vi "PicoLog1000ExampleStreaming.vi"(1 "stop":bool) -> ()   [LabVIEW 2010]
panel:
  out "UnitInfo":T1
  out "maxValue":u16
  in  "Apply":bool
  in  "Duty Cycle (%)":u8 max=100
  in  "Period (microseconds)":u16=100 min=100 max=1800
  in  "D3":bool=TRUE
  in  "D2":bool=TRUE
  in  "D1":bool=TRUE
  in  "D0":bool=TRUE
  in  "Trigger":T2={"Enabled"=FALSE, "AutoTrigger"=FALSE, "delay (%)"=-50.0, "Auto Trigger\nTiime (ms)"=1000, "Channel"=1, "Trigger Direction"=0, "threshold (mV)"=500, "hysteresis (mV)"=5} {"Trigger Direction" items=["rising edge", "falling edge"]; "Channel" items=["Ch1"=1, "Ch2"=2, "Ch3"=3, "Ch4"=4, "Ch5"=5, "Ch6"=6, "Ch7"=7, "Ch8"=8, "Ch9"=9, "Ch10"=10, "Ch11"=11, "Ch12"=12, "Ch13"=13, "Ch14"=14, "Ch15"=15, "Ch16"=16]}
  out "Ch Over Range":bool[](array[boolean])
  out "Ready":bool
  out "pl1000 handle out":i16
  out "error out":errorcluster
  in  "error in (no error)":errorcluster
  out "noOfValues":u32
  out "Triggered":bool
  out "Sampling rate (S/s)":dbl
  out "No. of channels":i16=12
  in  "Channels Enabled":string="1,2,3,4,5,6,7,8,9,10,11,12"
  out "Waveform Chart":dbl[][](graph)
  in  "Desired sample rate (S/s)":u32=2000 max=100000
  # "Streaming Mode Example"
  # "(e.g. 1,2,3)"
  # "Digital Outputs"
  # "Pulse-Width Modulation"
  # "OFF"
  # "ON"
  # "Trigger delay of \n-50% means the\ntrigger event is\nin the middle of \nthe block"
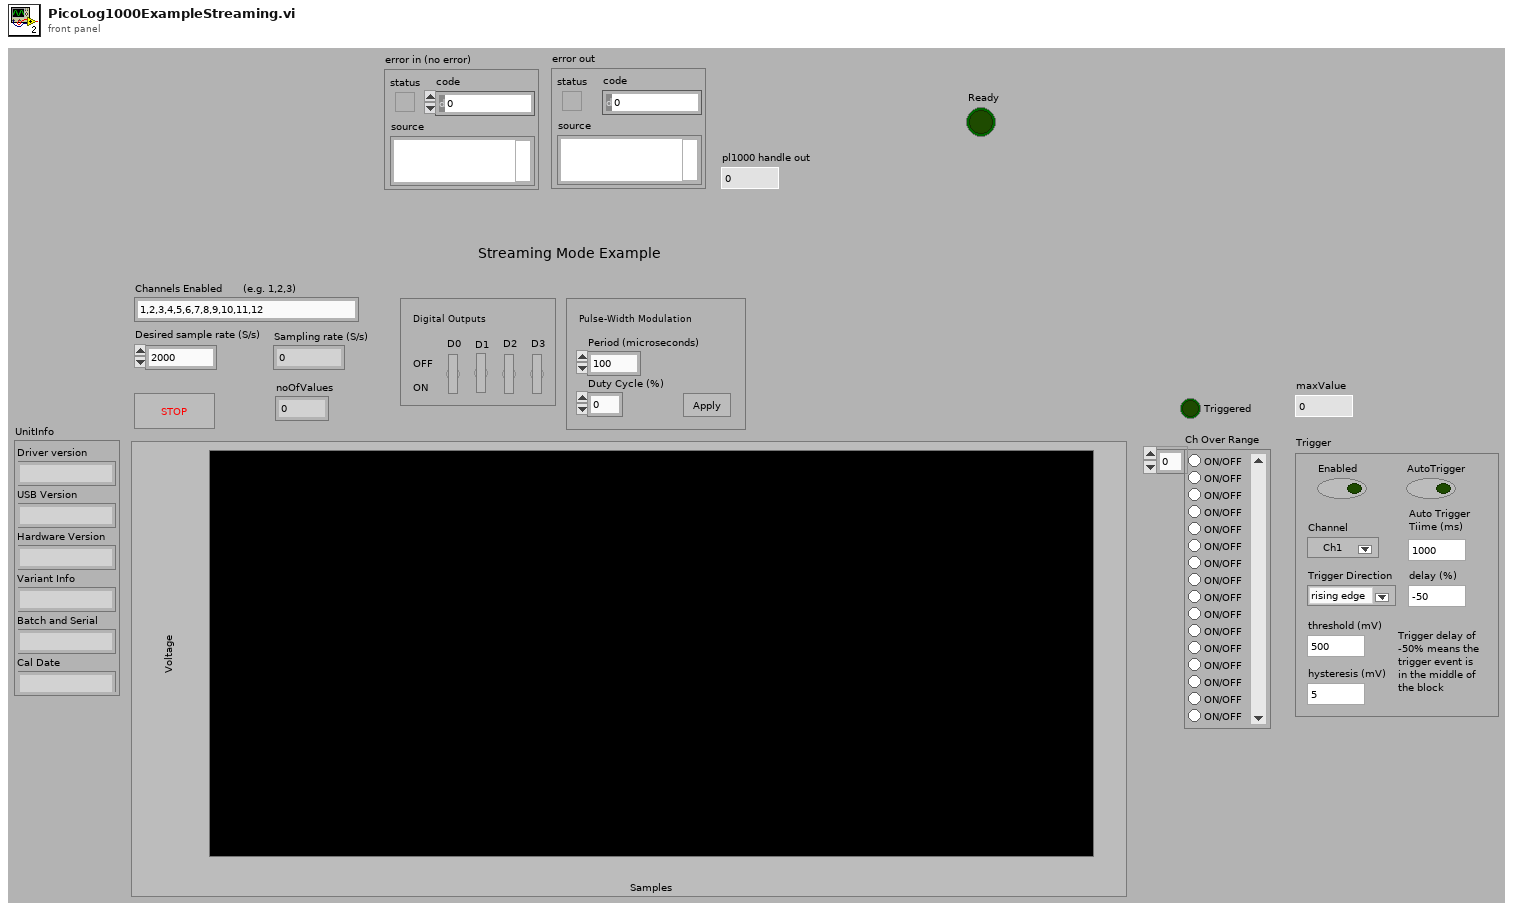
[diagram p1: front panel]
types:
  T1 = cluster{"Driver version":string, "USB Version":string, "Hardware Version":string, "Variant Info":string, "Batch and Serial":string, "Cal Date":string, "[6]":string, "[7]":string, "[8]":string}
  T2 = cluster{"Enabled":bool, "AutoTrigger":bool, "delay (%)":sgl, "Auto Trigger\nTiime (ms)":u16, "Channel":u16, "Trigger Direction":u16, "threshold (mV)":u16, "hysteresis (mV)":u16}
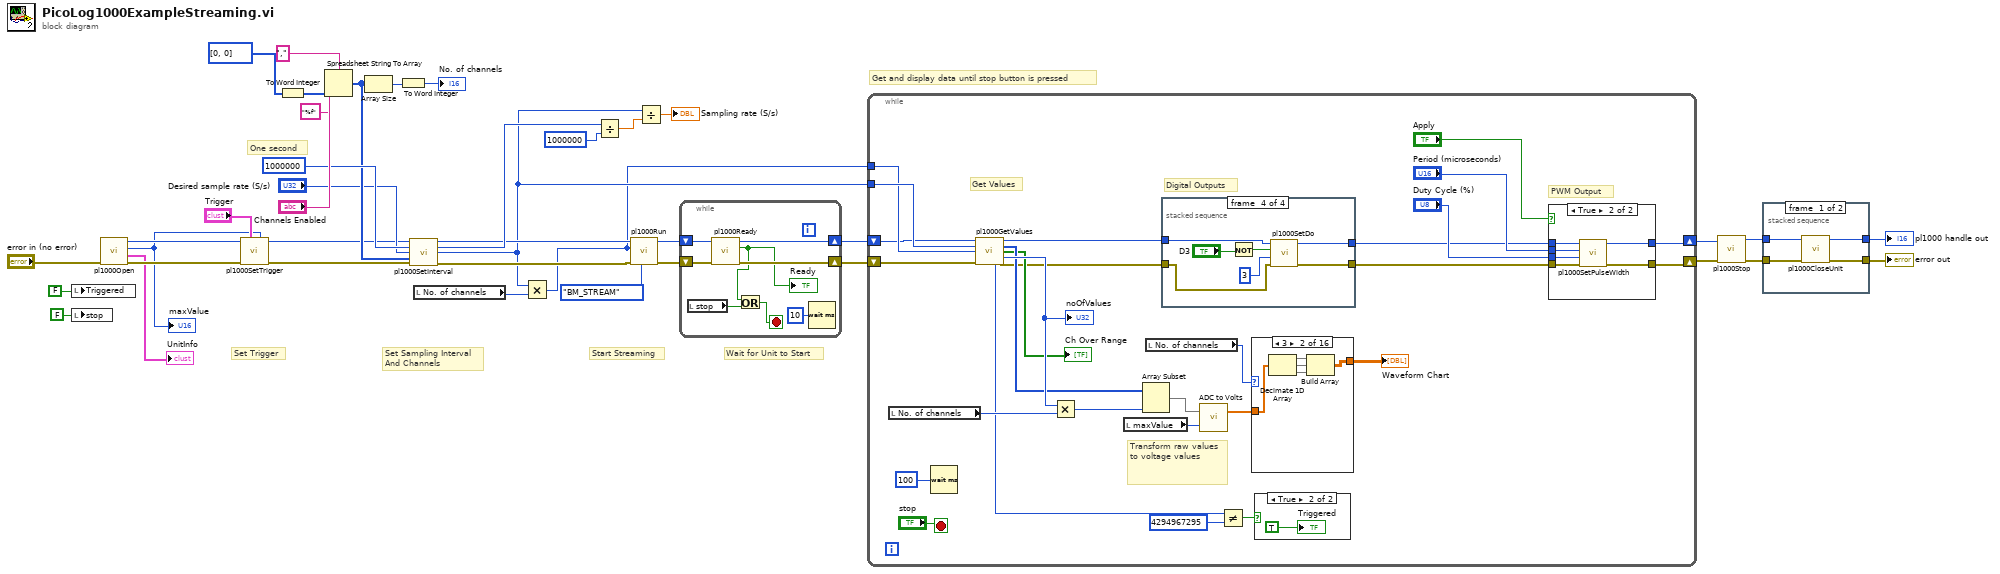
[diagram p0: block diagram]
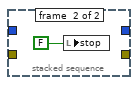
[diagram p2: hidden frame]
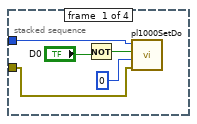
[diagram p4: hidden frame]
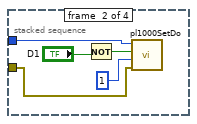
[diagram p5: hidden frame]
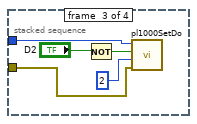
[diagram p6: hidden frame]
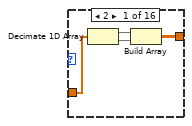
[diagram p8: hidden frame]
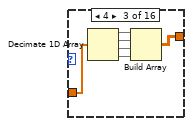
[diagram p9: hidden frame]
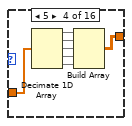
[diagram p10: hidden frame]
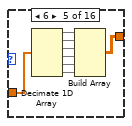
[diagram p11: hidden frame]
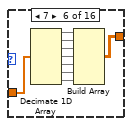
[diagram p12: hidden frame]
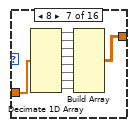
[diagram p13: hidden frame]
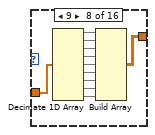
[diagram p14: hidden frame]
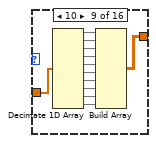
[diagram p15: hidden frame]
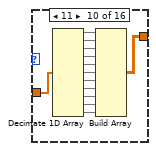
[diagram p16: hidden frame]
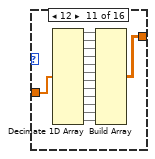
[diagram p17: hidden frame]
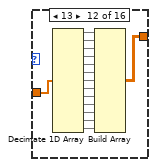
[diagram p18: hidden frame]
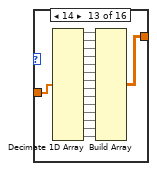
[diagram p19: hidden frame]
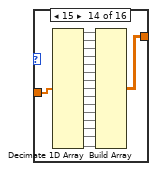
[diagram p20: hidden frame]
diagram:
  # "Wait for Unit to Start"
  # "Start Streaming"
  # "Set Sampling Interval\nAnd Channels"
  # "Set Trigger"
  # "Get and display data until stop button is pressed"
  # "One second"
  n1 = local write "Triggered"(FALSE ("Boolean")) -> ()
  n2 = local write "stop"(FALSE ("stop")) -> ()
  n3 = call "pl1000Open.vi"("error in (no error)"="error in (no error)") -> ("error out"=w11:errorcluster, "UnitInfo"=→"UnitInfo":T1, "maxValue"=w2:u16, "pl1000 handle out"=w7:i16)  [unwired: 7 in]
  "maxValue" <- w2
  n4 = call "pl1000SetTrigger.vi"("pl1000 handle"=w7, "Trigger"="Trigger", "maxValue"=w2, "error in (no error)"=w11) -> ("pl1000 handle out"=w9:i16, "error out"=w10:errorcluster)  [unwired: 10 in]
  n5 = To Word Integer(number=u32[] [0, 0] ("array type (2D Dbl)")) -> (16bit integer=w30:i16[])
  n6 = Spreadsheet String To Array(delimiter (Tab)=",", format string="%f", spreadsheet string="Channels Enabled", array type (2D Dbl)=w30) -> (array=w26:i16[])
  n7 = Array Size(array=w26) -> (size(s)=w32:i32)
  n8 = To Word Integer(number=w32) -> (16bit integer=→"No. of channels":i16)
  n9 = call "pl1000SetInterval.vi"("pl1000 handle"=w9, "usForBlock"=u32 1000000 ("us_for_block"), "idealNoOfSamples"="Desired sample rate (S/s)", "channels"=w26, "error in (no error)"=w10) -> ("pl1000 handle out"=w22:i16, "usForBlock OP"=w25:u32, "idealNoOfSamples OP"=w17:u32, "error out"=w23:errorcluster)  [unwired: 7 in]
  n10 = local read "No. of channels"() -> (w35:i16)
  n11 = Multiply(x=w17, y=w35) -> (x*y=w16:u32)
  n12 = Divide(x=w25, y=u32 1000000) -> (x/y=w36:dbl)
  n13 = call "pl1000Run.vi"("method"=enum16{"BM_SINGLE", "BM_WINDOW", "BM_STREAM"}."BM_STREAM", "error in (no error)"=w23, "noOfValues"=w16, "pl1000 handle"=w22) -> ("error out"=w20:errorcluster, "pl1000 handle out"=w19:i16)  [unwired: 6 in]
  n14 = Divide(x=w17, y=w36) -> (x/y=→"Sampling rate (S/s)":dbl)
  n15 = while {
    shift-right: [w46] -> w18
    shift-left: w19 -> [w48]
    shift-right: [w45] -> w15
    shift-left: w20 -> [w47]
    stop <- w43 stop-if-true
    n16 = local read "stop"() -> (w41:bool)
    n17 = call "pl1000Ready.vi"("error in (no error)"=w47, "pl1000 handle"=w48) -> ("error out"=w45:errorcluster, "ready"=w42:bool, "pl1000 handle out"=w46:i16)  [unwired: 7 in]
    "Ready" <- w42
    n18 = Or(x=w42, y=w41) -> (x .or. y?=w43:bool)
    n19 = Wait (ms)(milliseconds to wait=u32 10) -> ()  [unwired: 1 out]
  }
  n20 = while {
    tunnel: w17 -> [w66]
    tunnel: w16 -> [w65]
    shift-right: [w51] -> w13
    shift-left: w15 -> [w61]
    shift-right: [w50] -> w12
    shift-left: w18 -> [w59]
    stop <- "stop" stop-if-true
    # "Transform raw values to voltage values"
    # "Get Values"
    # "PWM Output"
    # "Digital Outputs"
    n21 = local read "No. of channels"() -> (w73:i16)
    n22 = Wait (ms)(milliseconds to wait=u32 100) -> ()  [unwired: 1 out]
    n23 = call "pl1000GetValues.vi"("pl1000 handle"=w59, "noOfValues"=w66, "SizeOfArray"=w65, "error in (no error)"=w61) -> ("pl1000 handle out"=w58:i16, "values"=w67:u16[], "Ch Over Range"=→"Ch Over Range":bool[], "noOfValues collected per ch"=w68:u32, "triggerIndex"=w64:u32, "error out"=w57:errorcluster)  [unwired: 6 in]
    "noOfValues" <- w68
    n24 = Multiply(x=w68, y=w73) -> (x*y=w72:u32)
    n25 = local read "maxValue"() -> (w49:u16)
    n26 = Array Subset(array=w67, length=w72) -> (w63:u16[])  [unwired: 1 in]
    n27 = local read "No. of channels"() -> (w75:i16)
    n28 = stacked-sequence {
      tunnel: w58 -> [w86 w91 w96 w103]
      tunnel: w57 -> [w85 w90 w95 w100]
      tunnel: [_ _ _ w101] -> w52
      tunnel: [_ _ _ w102] -> w53
      frame #0 {
        n29 = Not(x="D0") -> (.not. x?=w89:bool)
        n30 = call "pl1000SetDo.vi"("error in (no error)"=w85, "DO Channel"=0, "DO State"=w89, "pl1000 handle"=w86) -> ()  [unwired: 6 in, 2 out]
      }
      frame #1 {
        n31 = Not(x="D1") -> (.not. x?=w94:bool)
        n32 = call "pl1000SetDo.vi"("error in (no error)"=w90, "DO Channel"=1, "DO State"=w94, "pl1000 handle"=w91) -> ()  [unwired: 6 in, 2 out]
      }
      frame #2 {
        n33 = Not(x="D2") -> (.not. x?=w99:bool)
        n34 = call "pl1000SetDo.vi"("error in (no error)"=w95, "DO Channel"=2, "DO State"=w99, "pl1000 handle"=w96) -> ()  [unwired: 6 in, 2 out]
      }
      frame #3 {
        n35 = Not(x="D3") -> (.not. x?=w106:bool)
        n36 = call "pl1000SetDo.vi"("error in (no error)"=w100, "DO Channel"=3, "DO State"=w106, "pl1000 handle"=w103) -> ("error out"=w101:errorcluster, "pl1000 handle out"=w102:i16)  [unwired: 6 in]
      }
    }
    n37 = call "ADC to Volts.vi"("maxValue"=w49, "ADC values"=w63) -> ("values in Volt"=w62:dbl[])  [unwired: 1 in]
    n38 = Not Equal?(x=w64, y=u32 4294967295) -> (x != y?=w71:bool)
    n39 = case shown="3" w75 {
      tunnel: [w109 w114 w120 w127 w135 w144 w154 w165 w177 w190 w204 w219 w235 w252 w270 w274] -> w74
      tunnel: w62 -> [w108 w112 w117 w123 w130 w138 w147 w157 w168 w180 w193 w207 w222 w238 w255 w273]
      frame 2 {
        n40 = Decimate 1D Array(w108) -> (w111:dbl[], w110:dbl[])
        n41 = Build Array(w111, w110) -> (w109:dbl[][])
      }
      frame 3 {
        n42 = Decimate 1D Array(w112) -> (w116:dbl[], w115:dbl[], w113:dbl[])
        n43 = Build Array(w116, w115, w113) -> (w114:dbl[][])
      }
      frame 4 {
        n44 = Decimate 1D Array(w117) -> (w122:dbl[], w121:dbl[], w119:dbl[], w118:dbl[])
        n45 = Build Array(w122, w121, w119, w118) -> (w120:dbl[][])
      }
      frame 5 {
        n46 = Decimate 1D Array(w123) -> (w129:dbl[], w128:dbl[], w126:dbl[], w125:dbl[], w124:dbl[])
        n47 = Build Array(w129, w128, w126, w125, w124) -> (w127:dbl[][])
      }
      frame 6 {
        n48 = Decimate 1D Array(w130) -> (w137:dbl[], w136:dbl[], w134:dbl[], w133:dbl[], w132:dbl[], w131:dbl[])
        n49 = Build Array(w137, w136, w134, w133, w132, w131) -> (w135:dbl[][])
      }
      frame 7 {
        n50 = Decimate 1D Array(w138) -> (w146:dbl[], w145:dbl[], w143:dbl[], w142:dbl[], w141:dbl[], w140:dbl[], w139:dbl[])
        n51 = Build Array(w146, w145, w143, w142, w141, w140, w139) -> (w144:dbl[][])
      }
      frame 8 {
        n52 = Decimate 1D Array(w147) -> (w156:dbl[], w155:dbl[], w153:dbl[], w152:dbl[], w151:dbl[], w150:dbl[], w149:dbl[], w148:dbl[])
        n53 = Build Array(w156, w155, w153, w152, w151, w150, w149, w148) -> (w154:dbl[][])
      }
      frame 9 {
        n54 = Decimate 1D Array(w157) -> (w167:dbl[], w166:dbl[], w164:dbl[], w163:dbl[], w162:dbl[], w161:dbl[], w160:dbl[], w159:dbl[], w158:dbl[])
        n55 = Build Array(w167, w166, w164, w163, w162, w161, w160, w159, w158) -> (w165:dbl[][])
      }
      frame 10 {
        n56 = Decimate 1D Array(w168) -> (w179:dbl[], w178:dbl[], w176:dbl[], w175:dbl[], w174:dbl[], w173:dbl[], w172:dbl[], w171:dbl[], w170:dbl[], w169:dbl[])
        n57 = Build Array(w179, w178, w176, w175, w174, w173, w172, w171, w170, w169) -> (w177:dbl[][])
      }
      frame 11 {
        n58 = Decimate 1D Array(w180) -> (w192:dbl[], w191:dbl[], w189:dbl[], w188:dbl[], w187:dbl[], w186:dbl[], w185:dbl[], w184:dbl[], w183:dbl[], w182:dbl[], w181:dbl[])
        n59 = Build Array(w192, w191, w189, w188, w187, w186, w185, w184, w183, w182, w181) -> (w190:dbl[][])
      }
      frame 12 {
        n60 = Decimate 1D Array(w193) -> (w206:dbl[], w205:dbl[], w203:dbl[], w202:dbl[], w201:dbl[], w200:dbl[], w199:dbl[], w198:dbl[], w197:dbl[], w196:dbl[], w195:dbl[], w194:dbl[])
        n61 = Build Array(w206, w205, w203, w202, w201, w200, w199, w198, w197, w196, w195, w194) -> (w204:dbl[][])
      }
      frame 13 {
        n62 = Decimate 1D Array(w207) -> (w221:dbl[], w220:dbl[], w218:dbl[], w217:dbl[], w216:dbl[], w215:dbl[], w214:dbl[], w213:dbl[], w212:dbl[], w211:dbl[], w210:dbl[], w209:dbl[], w208:dbl[])
        n63 = Build Array(w221, w220, w218, w217, w216, w215, w214, w213, w212, w211, w210, w209, w208) -> (w219:dbl[][])
      }
      frame 14 {
        n64 = Decimate 1D Array(w222) -> (w237:dbl[], w236:dbl[], w234:dbl[], w233:dbl[], w232:dbl[], w231:dbl[], w230:dbl[], w229:dbl[], w228:dbl[], w227:dbl[], w226:dbl[], w225:dbl[], w224:dbl[], w223:dbl[])
        n65 = Build Array(w237, w236, w234, w233, w232, w231, w230, w229, w228, w227, w226, w225, w224, w223) -> (w235:dbl[][])
      }
      frame 15 {
        n66 = Decimate 1D Array(w238) -> (w254:dbl[], w253:dbl[], w251:dbl[], w250:dbl[], w249:dbl[], w248:dbl[], w247:dbl[], w246:dbl[], w245:dbl[], w244:dbl[], w243:dbl[], w242:dbl[], w241:dbl[], w240:dbl[], w239:dbl[])
        n67 = Build Array(w254, w253, w251, w250, w249, w248, w247, w246, w245, w244, w243, w242, w241, w240, w239) -> (w252:dbl[][])
      }
      frame 16 {
        n68 = Decimate 1D Array(w255) -> (w272:dbl[], w271:dbl[], w269:dbl[], w268:dbl[], w267:dbl[], w266:dbl[], w265:dbl[], w264:dbl[], w263:dbl[], w262:dbl[], w261:dbl[], w260:dbl[], w259:dbl[], w258:dbl[], w257:dbl[], w256:dbl[])
        n69 = Build Array(w272, w271, w269, w268, w267, w266, w265, w264, w263, w262, w261, w260, w259, w258, w257, w256) -> (w270:dbl[][])
      }
      frame 1, Default {
        n70 = Decimate 1D Array(w273) -> (w275:dbl[])
        n71 = Build Array(w275) -> (w274:dbl[][])
      }
    }
    "Waveform Chart" <- w74
    n72 = case shown="True" w71 {
      frame False {
      }
      frame True {
        "Triggered" <- TRUE ("Boolean")
      }
    }
    n73 = case shown="True" "Apply" {
      tunnel: w53 -> [w77 w84]
      tunnel: "Period (microseconds)" -> [_ w83]
      tunnel: "Duty Cycle (%)" -> [_ w82]
      tunnel: w52 -> [w78 w81]
      tunnel: [w78 w80] -> w51
      tunnel: [w77 w79] -> w50
      frame False {
      }
      frame True {
        n74 = call "pl1000SetPulseWidth.vi"("error in (no error)"=w81, "cycle"=w82, "period"=w83, "pl1000 handle"=w84) -> ("error out"=w80:errorcluster, "pl1000 handle out"=w79:i16)  [unwired: 6 in]
      }
    }
  }
  n75 = call "pl1000Stop.vi"("error in (no error)"=w13, "pl1000 handle"=w12) -> ("error out"=w6:errorcluster, "pl1000 handle out"=w5:i16)  [unwired: 8 in]
  n76 = stacked-sequence {
    tunnel: w6 -> [w279 _]
    tunnel: w5 -> [w278 _]
    tunnel: [w277 _] -> w4
    tunnel: [w276 _] -> w3
    frame #0 {
      n77 = call "pl1000CloseUnit.vi"("error in (no error)"=w279, "pl1000 handle"=w278) -> ("error out"=w276:errorcluster, "pl1000 handle out"=w277:i16)  [unwired: 8 in]
    }
    frame #1 {
      n78 = local write "stop"(FALSE ("stop")) -> ()
    }
  }
  "error out" <- w3
  "pl1000 handle out" <- w4
